vi "example 5 - grand child.vi"() -> ()   [LabVIEW 2020]
panel:
  out "20?":bool
  in  "Double":dbl
  in  "Clear":bool
  in  "String":string
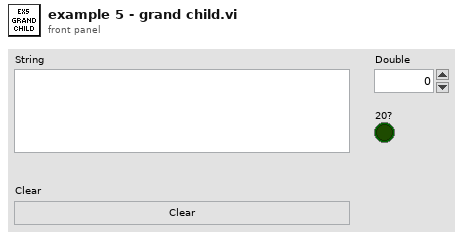
[diagram p1: front panel]
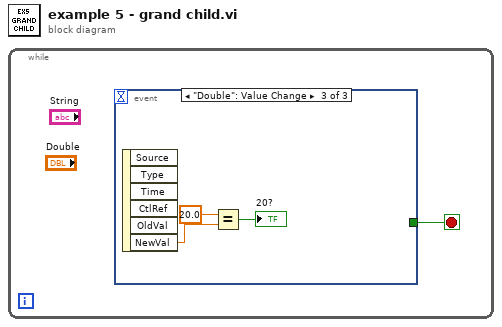
[diagram p0: block diagram]
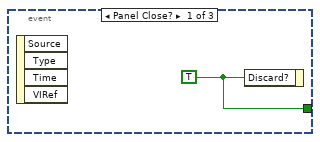
[diagram p2: hidden frame]
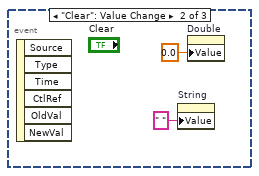
[diagram p3: hidden frame]
diagram:
  n1 = while {
    stop <- w1 stop-if-true
    n2 = event shown="[2] \"Double\": Value Change" {
      selector: _ -> [_ _ _]
      dyn-events: _ -> [_ _ _]
      timeout: _ -> [_ _ _]
      tunnel: [w2 _ _] -> w1
      event Panel Close? {
        w2 = TRUE
        n3 = event-data() -> ()  [unwired: 1 in, 4 out]
        n4 = event-data("Discard?"=w2) -> ()  [unwired: 1 in, 1 out]
      }
      event "Clear": Value Change {
        n5 = event-data() -> ()  [unwired: 1 in, 6 out]
        n6 = property on="String" class="Str"("Value"=" " ("String")) -> ()  [unwired: 2 in, 2 out]
        n7 = property on="Double" class="DigNum (strict)"("Value"=0.0 ("Double")) -> ()  [unwired: 2 in, 2 out]
      }
      event "Double": Value Change {
        n8 = event-data() -> ("NewVal"=w7:dbl)  [unwired: 1 in, 5 out]
        n9 = Equal?(x=20.0, y=w7) -> (x = y?=→"20?":bool)
      }
    }
  }
